vi "ODE Linear System Numeric.vi"(0 "X0 (start value)":dbl[](array[numeric]) format="%.2f", 1 "A (matrix of coefficients)":dbl[][](array[numeric]) format="%.2f", 2 "number of points":u32=10, 3 "time start":dbl format="%.2f", 4 "time end":dbl=1.0 format="%.2f") -> (5 "Times":dbl[](array[numeric]) format="%.2f", 6 "X Values":dbl[][](array[numeric]) format="%.2f", 7 "error":i32)   [LabVIEW 2020, in "NI_Gmath.lvlib"]
doc: "Solves an n-dimension, homogeneous linear system of differential equations with constant coefficients, for a given start condition."
uses:
  NI_Gmath.lvlib
  NI_AALPro.lvlib
  NI_AALBase.lvlib
  NI_Matrix.lvlib
panel:
  # "dX(t)/dt = AX(t)\nX(0) = X0"
  # "Example:\n\n A: ((1.0,2.0),(-2.3,1.1)) \n X0: 1.0 and 2.4 \n number of points: 100\n time start: 0.0 \n time end: 1.0"
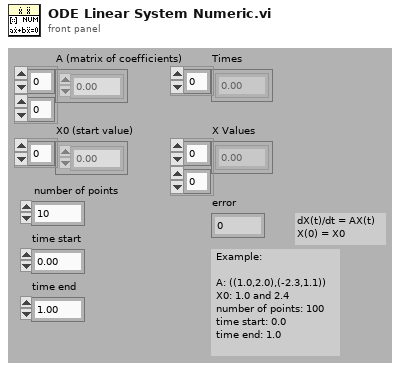
[diagram p1: front panel]
types:
  T1 = typedef "NI_Matrix.lvlib/ComplexMatrix.ctl" = cdb[][]
  T2 = typedef "NI_Matrix.lvlib/RealMatrix.ctl" = dbl[][]
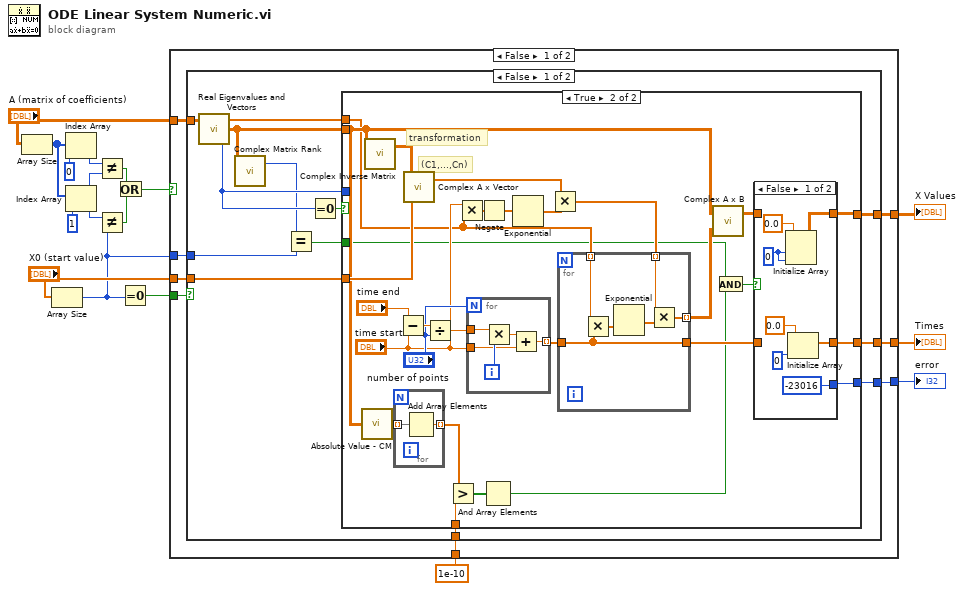
[diagram p0: block diagram]
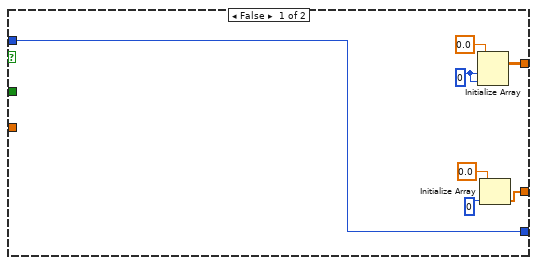
[diagram p2: hidden frame]
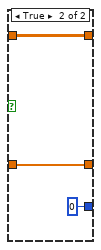
[diagram p3: hidden frame]
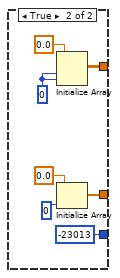
[diagram p4: hidden frame]
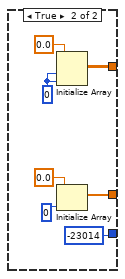
[diagram p5: hidden frame]
diagram:
  n1 = Array Size(array="A (matrix of coefficients)") -> (size(s)=w12:i32[])
  n2 = Array Size(array="X0 (start value)") -> (size(s)=w1:i32)
  n3 = Index Array(array=w12, index=0) -> (element=w14:i32)
  n4 = Index Array(array=w12, index=1) -> (element=w13:i32)
  n5 = Not Equal?(x=w14, y=w13) -> (x != y?=w11:bool)
  n6 = Not Equal?(x=w13, y=w1) -> (x != y?=w10:bool)
  n7 = Or(x=w11, y=w10) -> (x .or. y?=w9:bool)
  n8 = Equal To 0?(x=w1) -> (x = 0?=w7:bool)
  n9 = case shown="False" w9 {
    tunnel: [w23 -23014] -> w8
    tunnel: w7 -> [w24 _]
    tunnel: "A (matrix of coefficients)" -> [w22 _]
    tunnel: "X0 (start value)" -> [w21 _]
    tunnel: [w20 w104] -> w4
    tunnel: [w19 w103] -> w3
    tunnel: 1e-10 -> [w18 _]
    tunnel: w1 -> [w17 _]
    frame False {
      n10 = case shown="False" w24 {
        tunnel: [w37 -23013] -> w23
        tunnel: w22 -> [w31 _]
        tunnel: w21 -> [w36 _]
        tunnel: [w33 w97] -> w20
        tunnel: [w32 w96] -> w19
        tunnel: w18 -> [w29 _]
        tunnel: w17 -> [w25 _]
        frame False {
          n11 = call "Real Eigenvalues and Vectors.vi"("Input Matrix"=w31) -> ("error"=w35:i32, "Eigenvectors"=w28:T1, "Eigenvalues"=w30:cdb[])  [unwired: 2 in]
          n12 = call "Complex Matrix Rank.vi"("Input Matrix"=w28) -> ("rank"=w27:i32)  [unwired: 1 in, 1 out]
          n13 = Equal?(x=w27, y=w25) -> (x = y?=w26:bool)
          n14 = Equal To 0?(x=w35) -> (x = 0?=w34:bool)
          n15 = case shown="True" w34 {
            tunnel: w28 -> [_ w56]
            tunnel: w30 -> [_ w51]
            tunnel: w36 -> [_ w69]
            tunnel: [w43 w65] -> w37
            tunnel: w35 -> [w43 _]
            tunnel: [w42 w63] -> w33
            tunnel: [w38 w66] -> w32
            tunnel: w29 -> [_ w59]
            tunnel: w26 -> [_ w45]
            frame False {
              w39 = 0
              n16 = Initialize Array(0.0, w39, w39) -> (w42:dbl[][])
              n17 = Initialize Array(0.0, 0) -> (w38:dbl[])
            }
            frame True {
              # "(C1,...,Cn)"
              # "transformation"
              n18 = call "Absolute Value - CM.vi"("Complex Matrix A"=w56) -> ("|A|"=w60:T2)
              n19 = call "Complex Inverse Matrix.vi"("Input Matrix"=w56) -> ("Inverse Matrix"=w68:T1)  [unwired: 1 in, 1 out]
              n20 = for {
                tunnel: w60 -> [w79] mode=indexing
                tunnel: [w78] -> w61 mode=indexing
                n21 = Add Array Elements(numeric array=w79) -> (sum=w78:dbl)
              }
              n22 = Subtract(x="time end", y="time start") -> (x-y=w71:dbl)
              n23 = call "Complex A x Vector.vi"("Vector"=w69, "A"=w68) -> ("A x Vector"=w49:cdb[])  [unwired: 1 out]
              n24 = Divide(x=w71, y="number of points") -> (x/y=w54:dbl)
              n25 = Greater?(x=w61, y=w59) -> (0:w62:bool[])
              n26 = Multiply(x="time start", y=w51) -> (x*y=w50:cdb[])
              n27 = for {
                N: "number of points" -> [_]
                tunnel: "time start" -> [w75]
                tunnel: [w74] -> w53 mode=indexing
                tunnel: w54 -> [w73]
                i -> [w77]
                n28 = Multiply(x=w73, y=w77) -> (x*y=w76:dbl)
                n29 = Add(x=w76, y=w75) -> (x+y=w74:dbl)
              }
              n30 = Negate(x=w50) -> (-x=w46:cdb[])
              n31 = And Array Elements(Boolean array=w62) -> (logical AND=w58:bool)
              n32 = Exponential(1:w46) -> (0:w48:cdb[])
              n33 = Multiply(x=w49, y=w48) -> (x*y=w47:cdb[])
              n34 = for {
                tunnel: w51 -> [w95] mode=indexing
                tunnel: w47 -> [w93] mode=indexing
                tunnel: [w91] -> w72 mode=indexing
                tunnel: [w90] -> w67
                tunnel: w53 -> [w90]
                n35 = Multiply(x=w95, y=w90) -> (x*y=w94:cdb[])
                n36 = Exponential(1:w94) -> (0:w92:cdb[])
                n37 = Multiply(x=w93, y=w92) -> (x*y=w91:cdb[])
              }
              n38 = call "Complex A x B.vi"("B"=w72, "A"=w56) -> ("A x B"=w64:T1)  [unwired: 1 out]
              n39 = And(x=w45, y=w58) -> (x .and. y?=w57:bool)
              n40 = case shown="False" w57 {
                tunnel: w67 -> [_ w89]
                tunnel: [w81 w89] -> w66
                tunnel: [-23016 0] -> w65
                tunnel: w64 -> [_ w87]
                tunnel: [w82 w87] -> w63
                frame False {
                  w85 = 0
                  n41 = Initialize Array(0.0, w85, w85) -> (w82:dbl[][])
                  n42 = Initialize Array(0.0, 0) -> (w81:dbl[])
                }
                frame True {
                }
              }
            }
          }
        }
        frame True {
          w98 = 0
          n43 = Initialize Array(0.0, w98, w98) -> (w97:dbl[][])
          n44 = Initialize Array(0.0, 0) -> (w96:dbl[])
        }
      }
    }
    frame True {
      w105 = 0
      n45 = Initialize Array(0.0, w105, w105) -> (w104:dbl[][])
      n46 = Initialize Array(0.0, 0) -> (w103:dbl[])
    }
  }
  "error" <- w8
  "X Values" <- w4
  "Times" <- w3
